vi "set_wavelength.vi"(8 "error in (no error)":errorcluster, 10 "wavelength in":dbl[unit], 11 "LightSourceMH110124MaiTai in":refnum<class "LightSourceMH110124MaiTai.lvclass">) -> (0 "error out":errorcluster, 3 "LightSourceMH110124MaiTai out":refnum<class "LightSourceMH110124MaiTai.lvclass">)   [LabVIEW 2010, in "LightSourceMH110124MaiTai.lvclass"]
uses:
  LightSourceMH110124MaiTai.lvclass
  LightSourceMH110124MaiTai.lvclass/LightSourceMH110124MaiTai.ctl
  class_data.vi
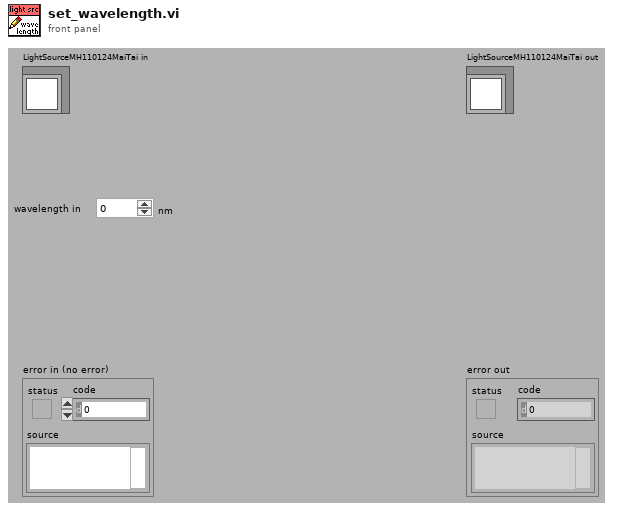
[diagram p1: front panel]
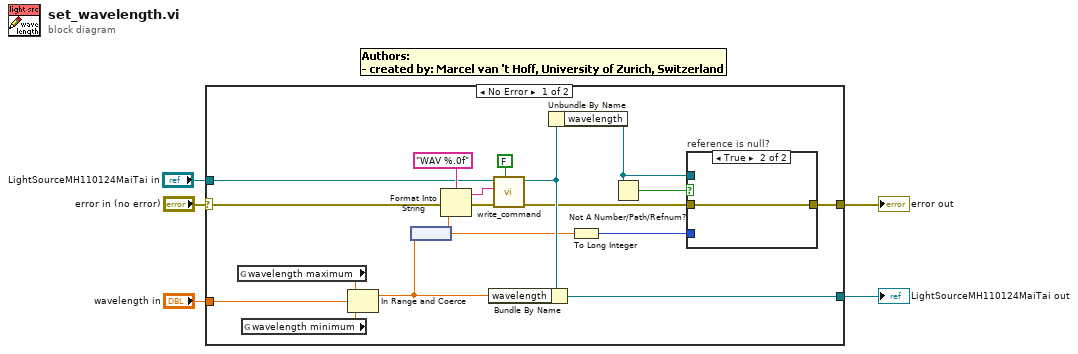
[diagram p0: block diagram]
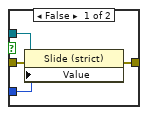
[diagram p2: hidden frame]
diagram:
  n1 = case shown="No Error" "error in (no error)" {
    selector: "error in (no error)" -> [w7 w30]
    tunnel: [w12 w30] -> w2
    tunnel: [w19 w29] -> w1
    tunnel: "LightSourceMH110124MaiTai in" -> [w6 w29]
    tunnel: "wavelength in" -> [w18 _]
    frame No Error {
      n2 = global read "class_data.vi" "wavelength maximum"() -> (w17:dbl[unit])
      n3 = global read "class_data.vi" "wavelength minimum"() -> (w16:dbl[unit])
      n4 = In Range and Coerce(upper limit=w17, x=w18, lower limit=w16) -> (coerced(x)=w15:dbl[unit])  [unwired: 1 out]
      n5 = node(w15) -> (w11:dbl)
      n6 = Format Into String(format string="WAV %.0f", error in=w7, w11) -> (resulting string=w21:string, error out=w23:errorcluster)  [unwired: 1 in]
      n7 = call-dynamic "write_command.vi"("read (T)"=FALSE, "error in (no error)"=w23, "string to write"=w21, "LightSourceMH110124MaiTai in"=w6) -> ("error out"=w13:errorcluster, "LightSourceMH110124MaiTai out"=w14:refnum<class "LightSourceMH110124MaiTai.lvclass">)  [unwired: 5 in, 1 out]
      n8 = Bundle By Name(cluster=w14, "wavelength"=w15) -> (w19:refnum<class "LightSourceMH110124MaiTai.lvclass">)
      n9 = Unbundle By Name(w14) -> ("wavelength"=w8:refnum<vi>)
      n10 = To Long Integer(number=w11) -> (32bit integer=w10:i32)
      n11 = Not A Number/Path/Refnum?(number/path/refnum=w8) -> (NaN/Path/Refnum?=w9:bool)
      n12 = case "reference is null?" shown="True" w9 {
        tunnel: w8 -> [w27 _]
        tunnel: w13 -> [w26 w28]
        tunnel: [w25 w28] -> w12
        tunnel: w10 -> [w24 _]
        frame False {
          n13 = property class="Slide (strict)"(reference=w27, error in=w26, "Value"=w24) -> (error out=w25:errorcluster)  [unwired: 1 out]
        }
        frame True {
        }
      }
    }
    frame Error {
    }
  }
  "error out" <- w2
  "LightSourceMH110124MaiTai out" <- w1
